vi "SmartSEM Remote API FIB VI slope.vi"(8 "error in":errorcluster, 11 "Api":refnum<k7>(container)) -> (0 "error out":errorcluster, 2 "V/I slope":sgl format="%.1g", 3 "Api out":refnum<k7>)   [LabVIEW 2018]
panel:
  in  "Cancel":bool
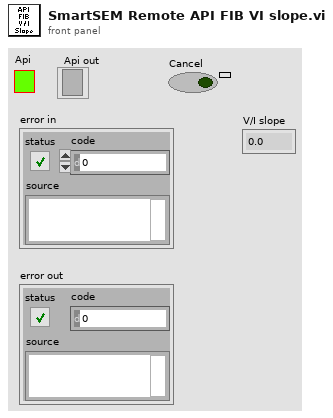
[diagram p1: front panel]
types:
  T1 = cluster{"Filament (A)":sgl, "Accelerator Target (V)":sgl, "Accelerator Actual (V)":sgl, "Extrator Target (V)":sgl, "Extrator Actual (V)":sgl, "Emission Target (uA)":sgl, "Emission Actual (uA)":sgl, "Suppressor (V)":sgl, "Faraday I (nA)":sgl, "Lens1 Target (V)":sgl, "Lens1 Actual (V)":sgl, "Lens2 Target (V)":sgl, "Lens2 Actual (V)":sgl, "Gun Vac (Torr)":sgl, "Column Vac (Torr)":sgl, "Tip Lifetime (uAhr)":sgl}
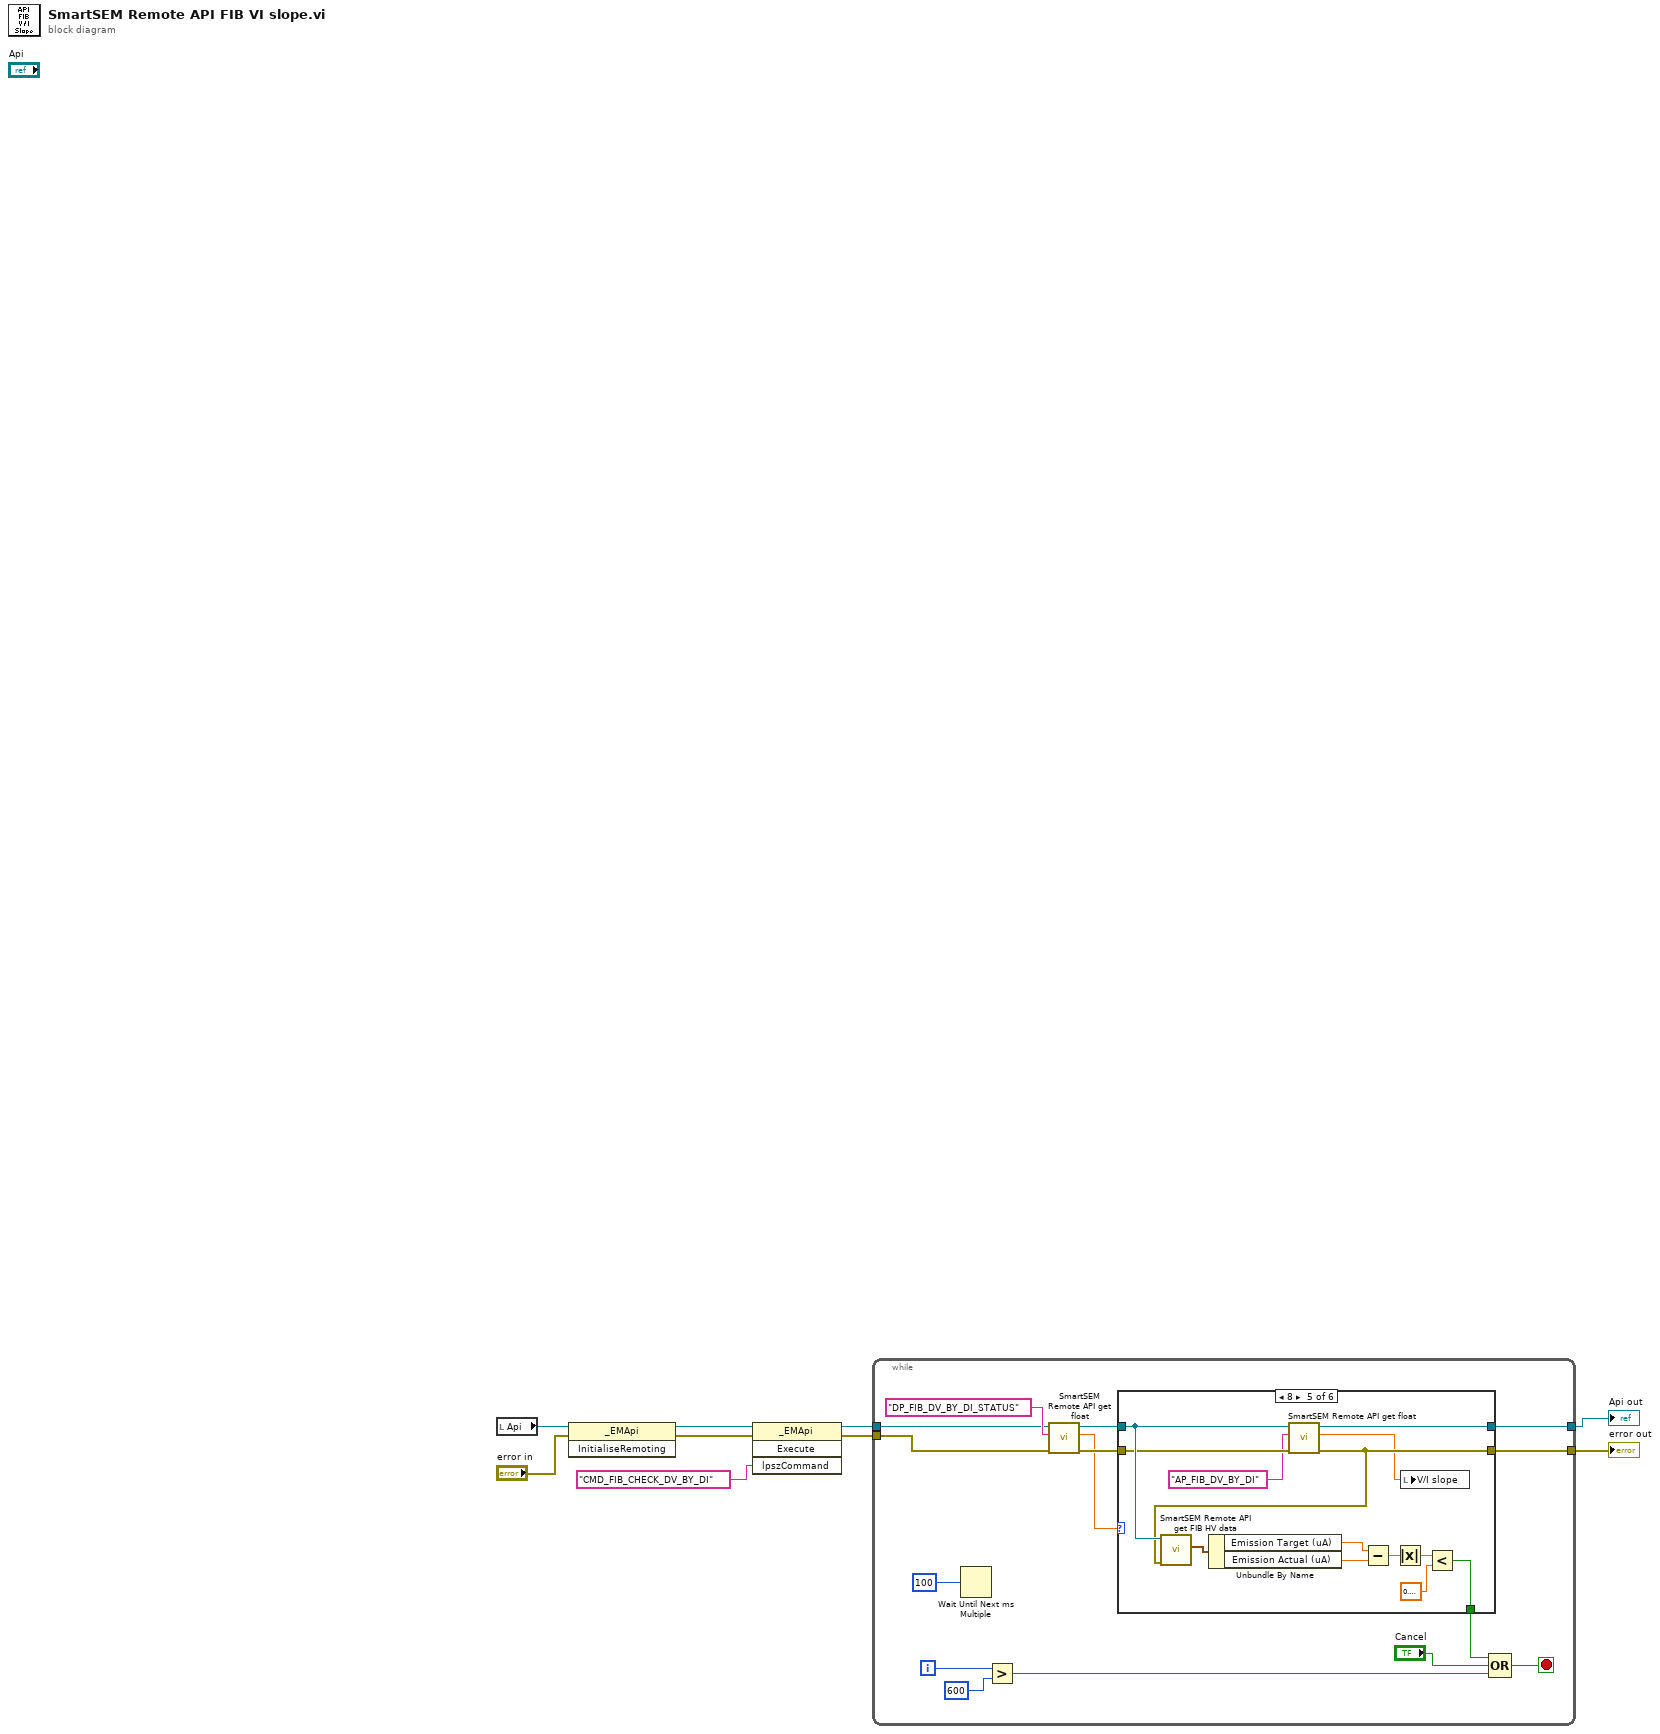
[diagram p0: block diagram]
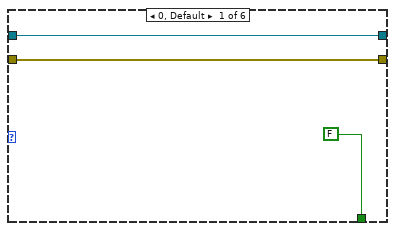
[diagram p2: hidden frame]
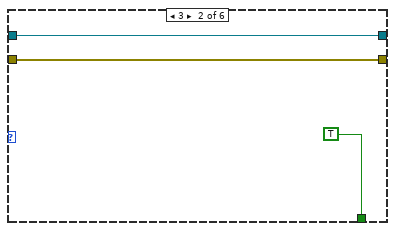
[diagram p3: hidden frame]
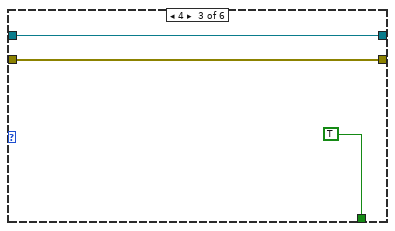
[diagram p4: hidden frame]
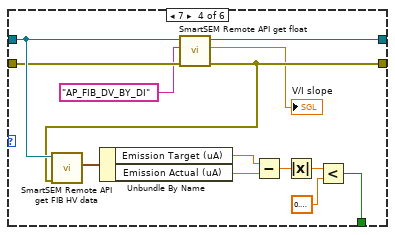
[diagram p5: hidden frame]
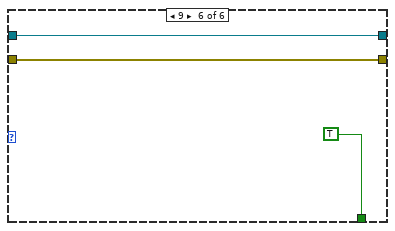
[diagram p6: hidden frame]
diagram:
  n1 = local read "Api"() -> (w9:refnum<k7>)
  n2 = invoke class="_EMApi" method="InitialiseRemoting"(reference=w9, error in="error in") -> (reference out=w7:refnum<k7>, error out=w6:errorcluster)  [unwired: 1 in, 1 out]
  n3 = invoke class="_EMApi" method="Execute"(reference=w7, error in=w6, "lpszCommand"="CMD_FIB_CHECK_DV_BY_DI") -> (reference out=w4:refnum<k7>, error out=w3:errorcluster)  [unwired: 1 in, 2 out]
  n4 = while {
    tunnel: w4 -> [w12]
    tunnel: w3 -> [w13]
    tunnel: [w24] -> w2
    tunnel: [w23] -> w1
    i -> [w18]
    stop <- w19 stop-if-true
    n5 = Wait Until Next ms Multiple(millisecond multiple=u32 100) -> ()  [unwired: 1 out]
    n6 = Greater?(x=w18, y=600) -> (0:w16:bool)
    n7 = call "SmartSEM Remote API get float.vi"("error in"=w13, "lpszParam"="DP_FIB_DV_BY_DI_STATUS" ("lpszCommand"), "Api"=w12) -> ("error out"=w14:errorcluster, "vValue"=w10:sgl, "Api out"=w11:refnum<k7>)  [unwired: 6 in]
    n8 = case shown="8" w10 {
      tunnel: [FALSE TRUE TRUE w43 w56 TRUE] -> w20
      tunnel: w11 -> [w26 w30 w33 w39 w52 w62]
      tunnel: [w26 w30 w33 w36 w49 w62] -> w24
      tunnel: w14 -> [w25 w29 w32 w38 w51 w61]
      tunnel: [w25 w29 w32 w37 w50 w61] -> w23
      frame 0, Default {
      }
      frame 3 {
      }
      frame 4 {
      }
      frame 7 {
        n9 = call "SmartSEM Remote API get float.vi"("error in"=w38, "lpszParam"="AP_FIB_DV_BY_DI" ("lpszCommand"), "Api"=w39) -> ("error out"=w37:errorcluster, "vValue"=→"V/I slope":sgl, "Api out"=w36:refnum<k7>)  [unwired: 6 in]
        n10 = call "SmartSEM Remote API get FIB HV data.vi"("error in"=w37, "Api in"=w39) -> ("Capella HV Data Output"=w40:T1)  [unwired: 6 in, 3 out]
        n11 = Unbundle By Name(w40) -> ("Emission Target (uA)"=w42:sgl, "Emission Actual (uA)"=w41:sgl)
        n12 = Subtract(x=w42, y=w41) -> (x-y=w46:sgl)
        n13 = Absolute Value(x=w46) -> (abs(x)=w45:sgl)
        n14 = Less?(x=w45, y=sgl 0.1) -> (x < y?=w43:bool)
      }
      frame 8 {
        n15 = call "SmartSEM Remote API get float.vi"("error in"=w51, "lpszParam"="AP_FIB_DV_BY_DI" ("lpszCommand"), "Api"=w52) -> ("error out"=w50:errorcluster, "vValue"=w47:sgl, "Api out"=w49:refnum<k7>)  [unwired: 6 in]
        n16 = call "SmartSEM Remote API get FIB HV data.vi"("error in"=w50, "Api in"=w52) -> ("Capella HV Data Output"=w53:T1)  [unwired: 6 in, 3 out]
        n17 = Unbundle By Name(w53) -> ("Emission Target (uA)"=w55:sgl, "Emission Actual (uA)"=w54:sgl)
        n18 = Subtract(x=w55, y=w54) -> (x-y=w59:sgl)
        n19 = Absolute Value(x=w59) -> (abs(x)=w58:sgl)
        n20 = local write "V/I slope"(w47) -> ()
        n21 = Less?(x=w58, y=sgl 0.1) -> (x < y?=w56:bool)
      }
      frame 9 {
      }
    }
    n22 = Compound Arithmetic op=OR(w20, "Cancel", w16) -> (w19:bool)
  }
  "Api out" <- w2
  "error out" <- w1
